vi "P3.3.vi"() -> ()   [LabVIEW 2020]
uses:
  <vilib>/Analysis/2dsp.llb/Real FFT.vi
  <vilib>/Analysis/2dsp.llb/Inverse Real FFT.vi
  <vilib>/Analysis/NI_AALPro.lvlib
panel:
  out "FFT":dbl[](graph)
  out "Imaginario":dbl[](graph)
  out "Real":dbl[](graph)
  out "Fase":dbl[](graph)
  out "Módulo":dbl[](graph)
  out "X 2":dbl[](array[numeric])
  out "X":dbl[](array[numeric])
  out "FFT {X}":cdb[](array[numeric])
  in  "FFT size":i32=-1
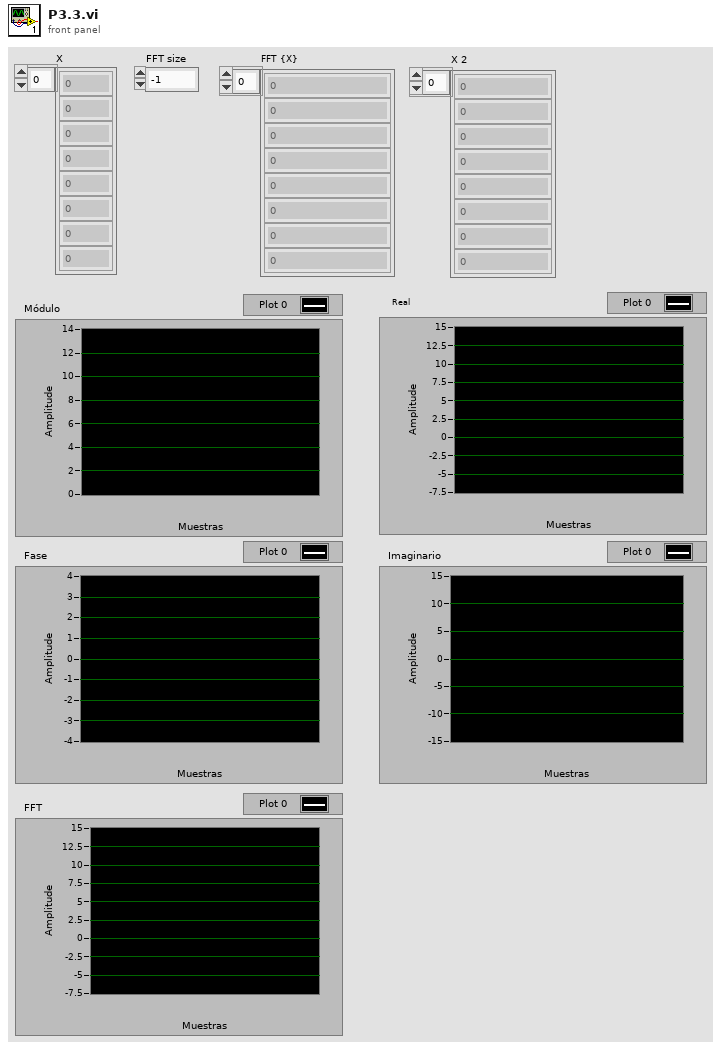
[diagram p1: front panel]
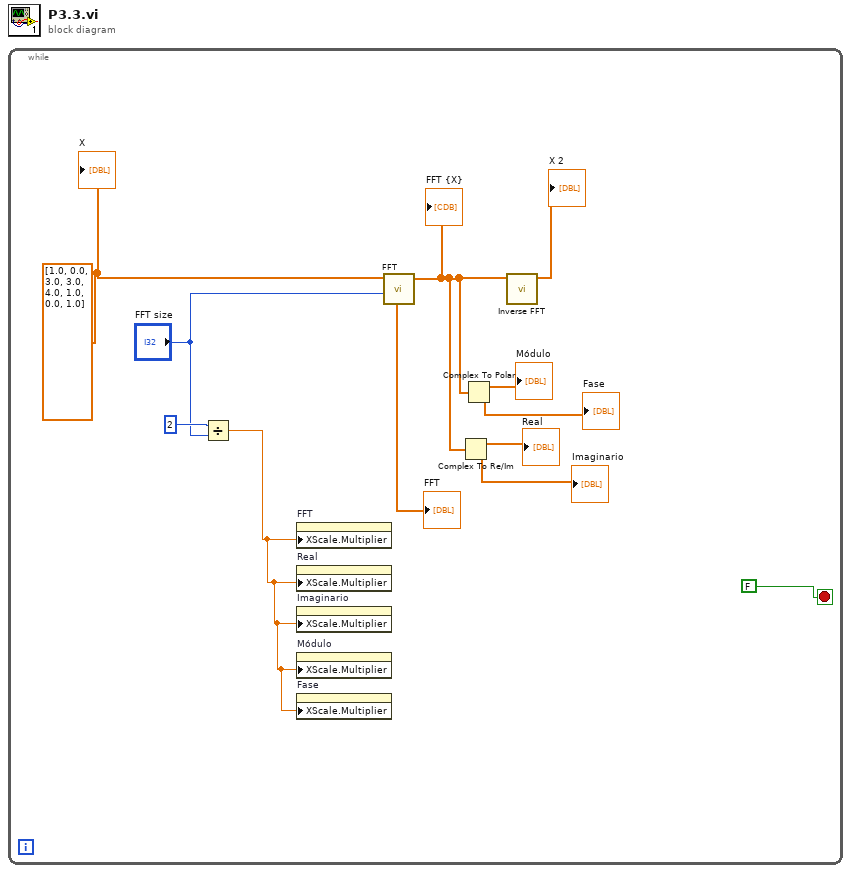
[diagram p0: block diagram]
diagram:
  n1 = while {
    stop <- FALSE ("stop") stop-if-true
    w11 = dbl[] [1.0, 0.0, 3.0, 3.0, 4.0, 1.0, 0.0, 1.0] ("X")
    n2 = Divide(x=2, y="FFT size") -> (x/y=w1:dbl)
    n3 = property on="FFT" class="WFGraph (strict)"("XScale.Multiplier"=w1) -> ()  [unwired: 2 in, 2 out]
    n4 = property on="Real" class="WFGraph (strict)"("XScale.Multiplier"=w1) -> ()  [unwired: 2 in, 2 out]
    n5 = property on="Imaginario" class="WFGraph (strict)"("XScale.Multiplier"=w1) -> ()  [unwired: 2 in, 2 out]
    n6 = property on="Módulo" class="WFGraph (strict)"("XScale.Multiplier"=w1) -> ()  [unwired: 2 in, 2 out]
    n7 = property on="Fase" class="WFGraph (strict)"("XScale.Multiplier"=w1) -> ()  [unwired: 2 in, 2 out]
    n8 = call-poly <vilib>:"FFT.vi"("FFT size"="FFT size", "X"=w11) -> ("FFT {X}"=w4:cdb[])  [unwired: 8 in, 1 out]
    "FFT {X}" <- w4
    "FFT" <- w4
    n9 = Complex To Re/Im(x + iy=w4) -> (x=→"Real":dbl[], y=→"Imaginario":dbl[])
    n10 = Complex To Polar(r * e^(i*theta)=w4) -> (r=→"Módulo":dbl[], theta=→"Fase":dbl[])
    n11 = call-poly <vilib>:"Inverse FFT.vi"("FFT {X}"=w4) -> ("X"=→"X 2":dbl[])  [unwired: 9 in, 1 out]
    "X" <- w11
  }
